vi "Workshop Exercise 4.vi"() -> ()   [LabVIEW 2019]
doc: "This VI demonstrates how to programmatically change the state of the front panel window. \n\nThere are six states that are related to the front panel of a VI; Standard, Maximize, Minimize, Hidden, Closed and Invalid. All states are read/write with the exception of Invalid, which is read only. The Standard state sets the VI to its default front panel state. The Maximize state will maximize the VI to full screen size. Minimize state is used to minimize the VI to the task bar. When using the Hidden state, the VI is still in memory, yet the front panel is hidden from view. The Closed state will also hide the front panel of the VI, but the front panel objects of the VI are no longer in memory. Lastly, the Invalid state is returned if an attempt is made to apply a window state at a time when it cannot be applied to the VI."
uses:
  <vilib>/Utility/miscctls.llb/LVRectTypeDef.ctl
panel:
  out "Device Temperature":dbl=35.02
  out "Voltage Alarm Level Exceeded?":bool=TRUE
  in  "Stop":bool
  # "You can place in here any additional controls and indicators needed for debugging"
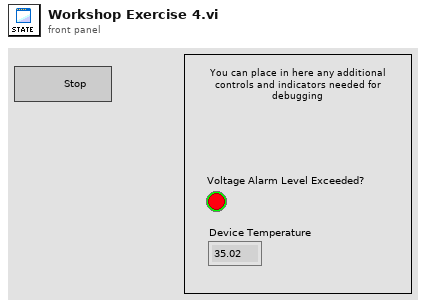
[diagram p1: front panel]
types:
  T1 = typedef "LVRectTypeDef.ctl" = cluster{"Left":i16, "Top":i16, "Right":i16, "Bottom":i16}
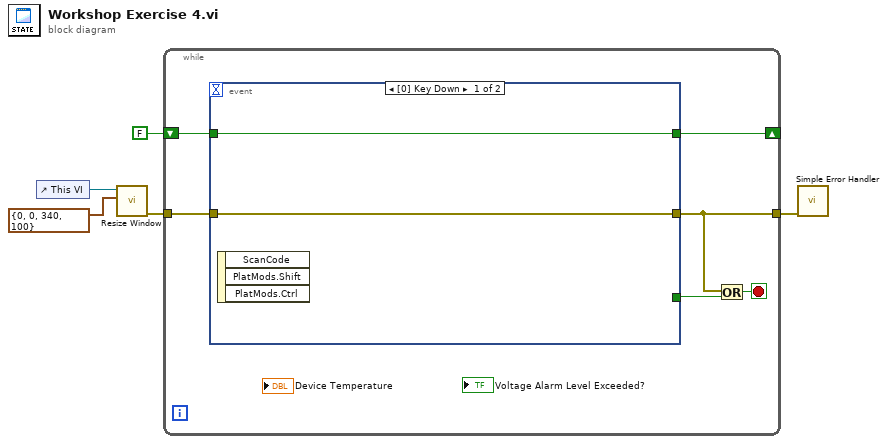
[diagram p0: block diagram]
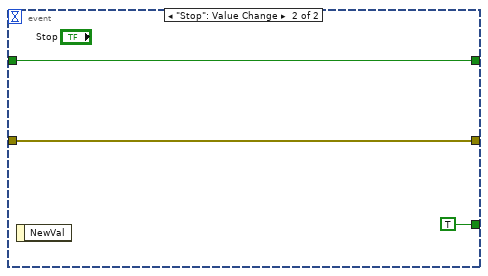
[diagram p2: hidden frame]
diagram:
  n1 = control-ref of="This VI"() -> (w3:refnum<vi>)
  n2 = call "Resize Window.vi"("Front Panel Window:Panel Bounds"=T1 {"Left"=0, "Top"=0, "Right"=340, "Bottom"=100}, "VI reference in"=w3) -> ("Error out"=w1:errorcluster)  [unwired: 8 in, 1 out]
  n3 = while {
    tunnel: [w9] -> w5
    tunnel: w1 -> [w8]
    shift-right: [w6] -> _
    shift-left: FALSE -> [w7]
    stop <- w10 stop-if-true
    # "Monitor User Interface Events"
    n4 = event shown="[0] Key Down" {
      selector: _ -> [_ _]
      dyn-events: _ -> [_ _]
      timeout: _ -> [_ _]
      tunnel: [_ TRUE ("T button?")] -> w11
      tunnel: [w12 w15] -> w9
      tunnel: w8 -> [w12 w15]
      tunnel: w7 -> [w13 w14]
      tunnel: [w13 w14] -> w6
      event Key Down {
        n5 = event-data() -> ()  [unwired: 4 out]
      }
      event "Stop": Value Change {
        # "Stop the VI."
        n6 = event-data() -> ()  [unwired: 2 out]
      }
    }
    n7 = Or(x=w9, y=w11) -> (x .or. y?=w10:bool)
  }
  n8 = call <vilib>:"Simple Error Handler.vi"("error in (no error)"=w5) -> ()  [unwired: 1 in, 8 out]
